vi "TEST - Tick Count (ms).vi"(8 "error in (no error)":errorcluster) -> (0 "error out":errorcluster, 2 "pass":bool)   [LabVIEW 2020]
uses:
  <vilib>/addons/_JKI Toolkits/Caraya/classes/Assert/Assert True.vi
  source/library/openg_time.lvlib
  <vilib>/addons/_JKI Toolkits/Caraya/classes/Test/Test.lvclass
  <vilib>/addons/_JKI Toolkits/Caraya/classes/Assert/Assert.lvclass
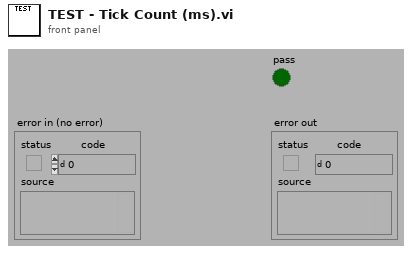
[diagram p1: front panel]
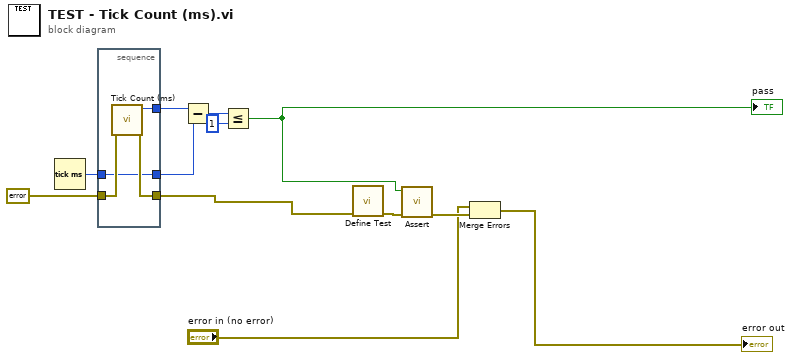
[diagram p0: block diagram]
diagram:
  n1 = Tick Count (ms)() -> (millisecond timer value=w10:u32)
  n2 = stacked-sequence {
    tunnel: [w16] -> w4
    tunnel: errorcluster {"status"=FALSE, "code"=0, "source"=""} ("error in (no error)") -> [w15]
    tunnel: [w14] -> w12
    tunnel: [w13] -> w11
    tunnel: w10 -> [w13]
    frame #0 {
      n3 = call "Tick Count (ms).vi"("error in (no error)"=w15) -> ("error out"=w16:errorcluster, "millisecond timer value"=w14:u32)  [unwired: 9 in]
    }
  }
  n4 = Subtract(x=w12, y=w11) -> (x-y=w9:u32)
  n5 = Less Or Equal?(x=w9, y=u32 1) -> (x <= y?=w5:bool)
  "pass" <- w5
  n6 = call <vilib>:"Define Test.vi"("error in (no error)"=w4) -> ("error out"=w6:errorcluster)  [unwired: 9 in, 1 out]
  n7 = call-poly <vilib>:"Assert.vi"("error in (no error)"=w6, "True?"=w5) -> ("error out"=w7:errorcluster)  [unwired: 8 in, 1 out]
  n8 = Merge Errors("error in (no error)", w7) -> (→"error out":errorcluster)
